vi "Tone-Compute Max Level.vi"(0 "Tone Params":T3, 9 "Level":T1, 11 "error in (no error)":errorcluster) -> (6 "Max Level":dbl, 10 "Level out":T1, 15 "error out":errorcluster)   [LabVIEW 2020]
uses:
  Tone Params.ctl
  Controls/Level XCtl/Level Data.ctl
  Controls/Level XCtl/Level Units.ctl
  Utility VIs/Math VIs/Linear to dB (scalar).vi
  PXI DAQ VIs/DAQ Engine VIs/PXI Globals.vi
  Controls/Level XCtl/Level XCtl.xctl
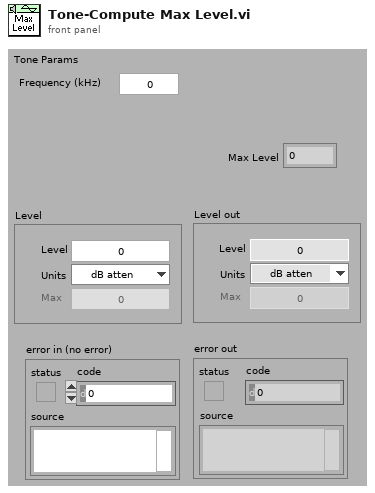
[diagram p1: front panel]
types:
  T1 = typedef "Level XCtl.xctl/Level Data.ctl" = cluster{"Level":dbl, "Units":T2, "Max":dbl, "Multiplier":dbl, "Cal File":path, "Cal":cluster{"Freq (Hz)":dbl[], "Mag (dB SPL)":dbl[], "Phase (deg)":dbl[]}}
  T2 = typedef "Level Units.ctl" = enum16{"dB atten", "dB SPL", "dB re 1 Vrms", "dB V/Hz½", "mW", "dB HL", "Volts", "dB mW"}
  T3 = typedef "Tone Params.ctl" = cluster{"Frequency (kHz)":dbl, "Last Freq":dbl, "Last Phase":dbl}
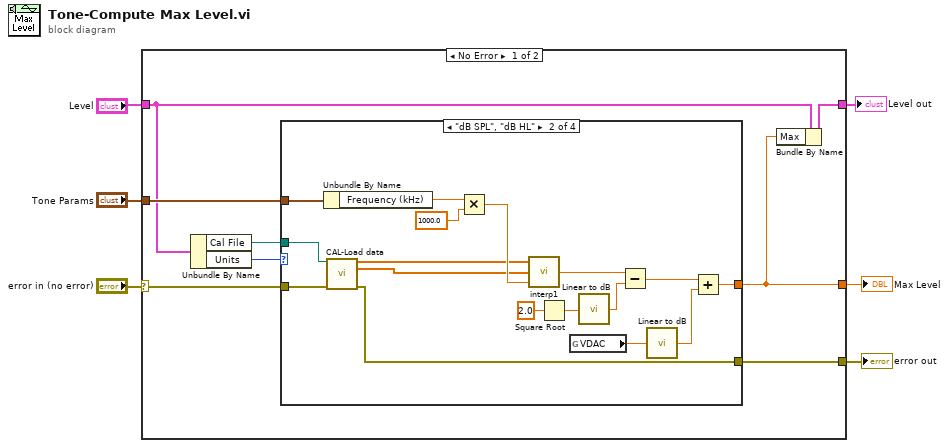
[diagram p0: block diagram]
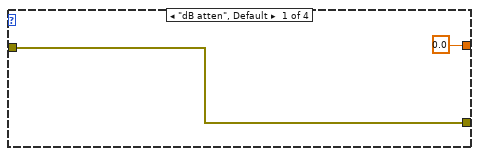
[diagram p2: hidden frame]
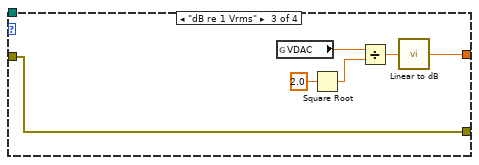
[diagram p3: hidden frame]
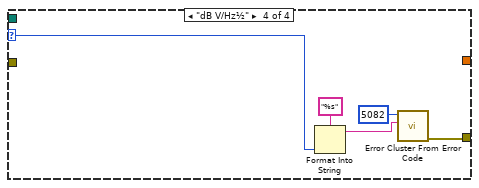
[diagram p4: hidden frame]
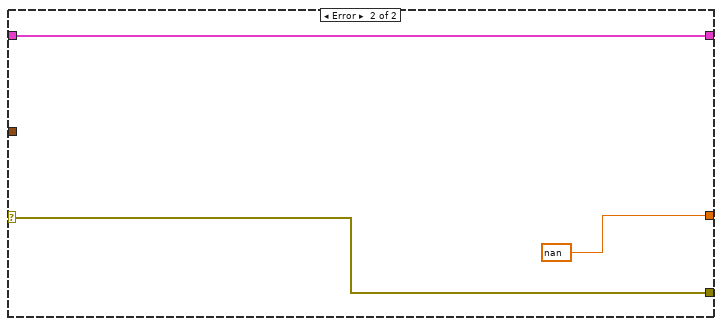
[diagram p5: hidden frame]
diagram:
  n1 = case shown="No Error" "error in (no error)" {
    selector: "error in (no error)" -> [w14 w47]
    tunnel: "Level" -> [w11 w45]
    tunnel: "Tone Params" -> [w13 _]
    tunnel: [w12 w47] -> w5
    tunnel: [w10 nan ("Reference Level")] -> w2
    tunnel: [w9 w45] -> w1
    frame No Error {
      n2 = Unbundle By Name(w11) -> ("Cal File"=w8:path, "Units"=w7:T2)
      n3 = case shown="\"dB SPL\", \"dB HL\"" w7 {
        selector: w7 -> [_ _ _ w40]
        tunnel: w14 -> [w15 w33 w39 _]
        tunnel: w13 -> [_ w24 _ _]
        tunnel: [0.0 ("Reference Level") w31 w34 _] -> w10
        tunnel: [w15 w20 w39 w41] -> w12
        tunnel: w8 -> [_ w19 _ _]
        frame "dB atten", Default {
        }
        frame "dB SPL", "dB HL" {
          n4 = Unbundle By Name(w24) -> ("Frequency (kHz)"=w29:dbl)
          n5 = call "CAL-Load data.vi"("user path"=w19, "error in (no error)"=w33) -> ("Frequency (Hz)"=w18:dbl[], "Mag"=w17:dbl[], "error out"=w20:errorcluster)  [unwired: 6 in, 5 out]
          n6 = Multiply(x=w29, y=1000.0) -> (x*y=w27:dbl)
          n7 = call "interp1.vi"("X"=w18, "Y"=w17, "U"=w27) -> ("V"=w25:dbl)  [unwired: 2 in]
          n8 = Square Root(x=2.0 ("y")) -> (sqrt(x)=w23:dbl)
          n9 = global read "PXI Globals.vi" "VDAC"() -> (w32:dbl)
          n10 = call-poly "Linear to dB.vi"("Linear"=w23) -> ("dB"=w22:dbl)
          n11 = Subtract(x=w25, y=w22) -> (x-y=w21:dbl)
          n12 = call-poly "Linear to dB.vi"("Linear"=w32) -> ("dB"=w30:dbl)
          n13 = Add(x=w21, y=w30) -> (x+y=w31:dbl)
        }
        frame "dB re 1 Vrms" {
          n14 = global read "PXI Globals.vi" "VDAC"() -> (w36:dbl)
          n15 = Square Root(x=2.0 ("y")) -> (sqrt(x)=w37:dbl)
          n16 = Divide(x=w36, y=w37) -> (x/y=w35:dbl)
          n17 = call-poly "Linear to dB.vi"("Linear"=w35) -> ("dB"=w34:dbl)
        }
        frame "dB V/Hz½" {
          n18 = Format Into String(format string="%s", w40) -> (resulting string=w43:string)  [unwired: 2 in, 1 out]
          n19 = call <vilib>:"Error Cluster From Error Code.vi"("error message (\"\")"=w43, "error code (0)"=5082) -> ("error out"=w41:errorcluster)  [unwired: 7 in]
        }
      }
      n20 = Bundle By Name(cluster=w11, "Max"=w10) -> (w9:T1)
    }
    frame Error {
    }
  }
  "error out" <- w5
  "Max Level" <- w2
  "Level out" <- w1
